vi "Get_Current_Scan_server.vi"(0 "Desired Channels":string[](array[string])) -> (1 "Ch Description Array":T1[](array[typedef]) {"Duty" format="%016b"; "D" format="%#_5g"; "C" format="%#_5g"; "B" format="%#_5g"; "A" format="%#_5g"}, 2 "String values":string[](array[string]), 3 "Numerical Values":dbl[](array[numeric]) format="%.2f")   [LabVIEW 2020]
uses:
  ADAM Client/Sub VIs/ADAM Controls/Ch_description_ADAM.ctl
  ADAM Client/Sub VIs/ADAM Controls/Module_type_ADAM.ctl
  ADAM Client/Sub VIs/ADAM Controls/Function_ADAM.ctl
  ADAM Client/Sub VIs/ADAM Controls/Channel_State.ctl
  ADAM Client/Sub VIs/ADAM Controls/Calib_type_ADAM.ctl
  ADAM Client/Sub VIs/ADAM Controls/Address.ctl
  ADAM_Global.vi
  Sub VI's/Channel_Description_Global.vi
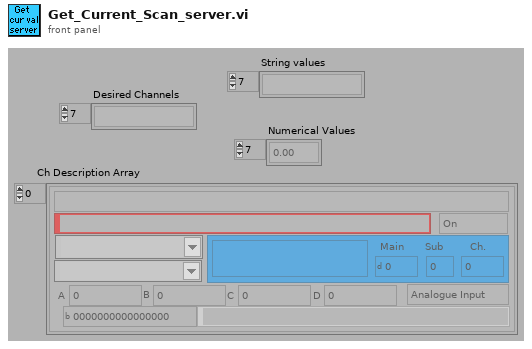
[diagram p1: front panel]
types:
  T1 = typedef "Ch_description_ADAM.ctl" = cluster{"Ch Name":string, "Type":T2, "Function":T3, "Ch State":T4, "Calibration type":T5, "A":dbl, "B":dbl, "C":dbl, "D":dbl, "Comments":string, "Address":T6, "String":string, "Duty":u16}
  T2 = typedef "Module_type_ADAM.ctl" = string
  T3 = typedef "Function_ADAM.ctl" = enum16{"Analogue Input", "Digital Input", "Event counter", "Event rate", "Analogue Output", "Digital Output", "Relay Output"}
  T4 = typedef "Channel_State.ctl" = enum16{"On", "Off", "Always On", "Always Off"}
  T5 = typedef "Calib_type_ADAM.ctl" = string
  T6 = typedef "Address.ctl" = cluster{"Main":i32, "Ch.":i32, "Sub":i32, "Port Name":string}
  T7 = typedef "Update_scan_value.ctl" = cluster{"Channel Name":string, "New Value":dbl}
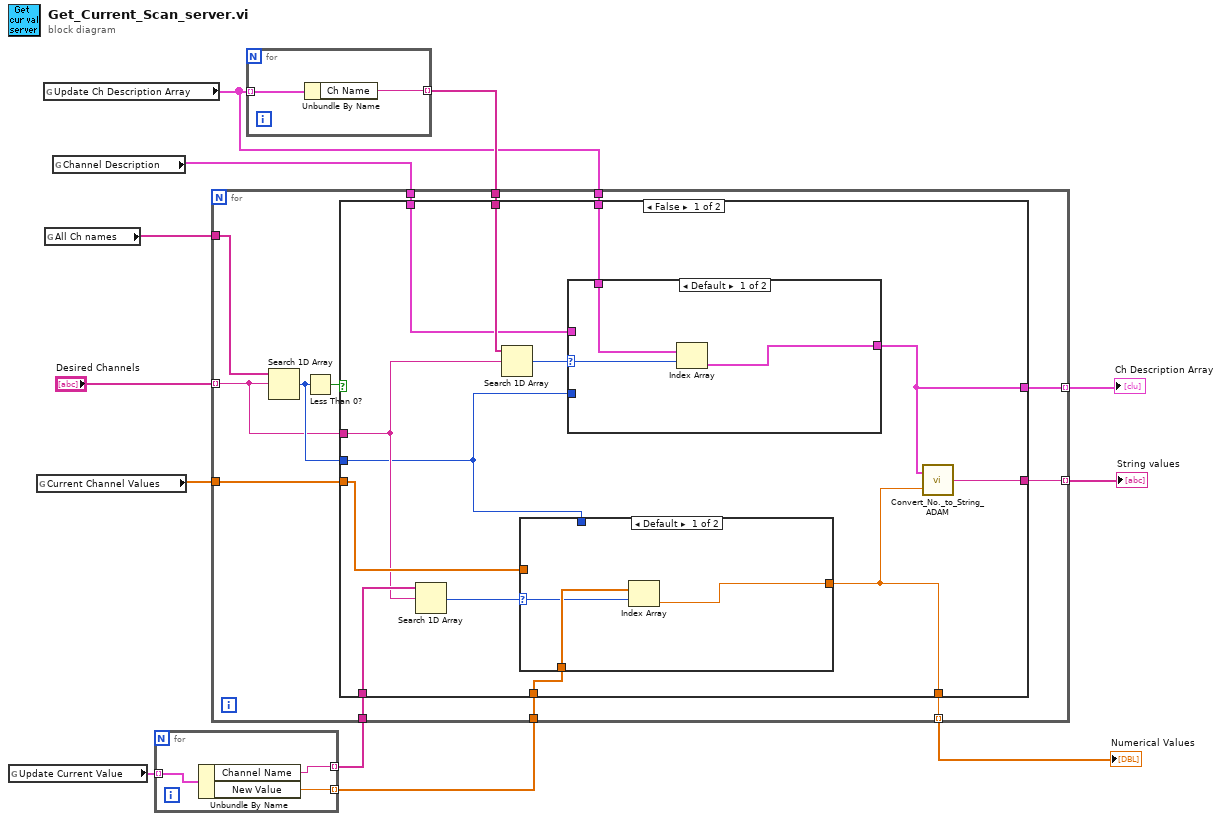
[diagram p0: block diagram]
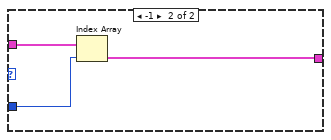
[diagram p2: hidden frame]
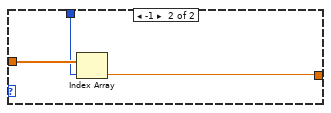
[diagram p3: hidden frame]
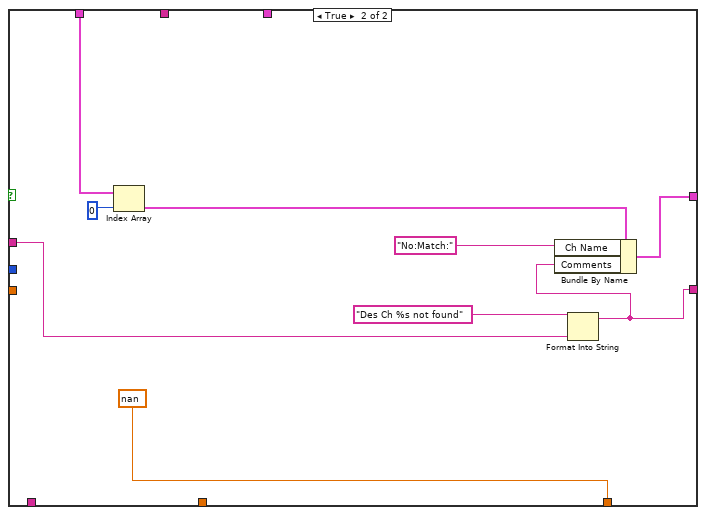
[diagram p4: hidden frame]
diagram:
  n1 = global read "ADAM_Global.vi" "Update Current Value"() -> (w5:T7[])
  n2 = global read "ADAM_Global.vi" "Current Channel Values"() -> (w11:dbl[])
  n3 = global read "ADAM_Global.vi" "Update Ch Description Array"() -> (w1:T1[])
  n4 = global read "ADAM_Global.vi" "All Ch names"() -> (w12:string[])
  n5 = global read "Channel_Description_Global.vi" "Channel Description"() -> (w6:T1[])
  n6 = for {
    tunnel: w5 -> [w15] mode=indexing
    tunnel: [w14] -> w4 mode=indexing
    tunnel: [w13] -> w3 mode=indexing
    n7 = Unbundle By Name(w15) -> ("Channel Name"=w14:string, "New Value"=w13:dbl)
  }
  n8 = for {
    tunnel: w1 -> [w17] mode=indexing
    tunnel: [w16] -> w2 mode=indexing
    n9 = Unbundle By Name(w17) -> ("Ch Name"=w16:string)
  }
  n10 = for {
    tunnel: "Desired Channels" -> [w22] mode=indexing
    tunnel: w12 -> [w30]
    tunnel: [w28] -> w10 mode=indexing
    tunnel: w11 -> [w26]
    tunnel: w6 -> [w25]
    tunnel: [w24] -> w9 mode=indexing
    tunnel: [w23] -> w7 mode=indexing
    tunnel: w4 -> [w21]
    tunnel: w3 -> [w20]
    tunnel: w2 -> [w19]
    tunnel: w1 -> [w18]
    n11 = Search 1D Array(1D array=w30, element=w22) -> (index of element=w27:i32)  [unwired: 1 out]
    n12 = Less Than 0?(x=w27) -> (x < 0?=w29:bool)
    n13 = case shown="False" w29 {
      tunnel: [w43 w56] -> w28
      tunnel: w27 -> [w33 _]
      tunnel: w26 -> [w40 _]
      tunnel: w25 -> [w34 w63]
      tunnel: [w39 nan] -> w24
      tunnel: [w31 w61] -> w23
      tunnel: w22 -> [w35 w58]
      tunnel: w21 -> [w42 _]
      tunnel: w20 -> [w38 _]
      tunnel: w19 -> [w36 _]
      tunnel: w18 -> [w32 _]
      frame False {
        n14 = Search 1D Array(1D array=w42, element=w35) -> (index of element=w41:i32)  [unwired: 1 out]
        n15 = Search 1D Array(1D array=w36, element=w35) -> (index of element=w37:i32)  [unwired: 1 out]
        n16 = case shown="Default" w41 {
          selector: w41 -> [w51 _]
          tunnel: w40 -> [_ w55]
          tunnel: w33 -> [_ w54]
          tunnel: [w50 w53] -> w39
          tunnel: w38 -> [w52 _]
          frame Default {
            n17 = Index Array(array=w52, index=w51) -> (element=w50:dbl)
          }
          frame -1 {
            n18 = Index Array(array=w55, index=w54) -> (element=w53:dbl)
          }
        }
        n19 = case shown="Default" w37 {
          selector: w37 -> [w46 _]
          tunnel: [w45 w49] -> w31
          tunnel: w34 -> [_ w48]
          tunnel: w33 -> [_ w47]
          tunnel: w32 -> [w44 _]
          frame Default {
            n20 = Index Array(array=w44, index=w46) -> (element=w45:T1)
          }
          frame -1 {
            n21 = Index Array(array=w48, index=w47) -> (element=w49:T1)
          }
        }
        n22 = call "Convert_No._to_String_ADAM.vi"("Input number"=w39, "Ch Description"=w31) -> ("Output sting"=w43:string)
      }
      frame True {
        n23 = Index Array(array=w63, index=0 ("Index")) -> (element=w62:T1)
        n24 = Format Into String(format string="Des Ch %s not found", w58) -> (resulting string=w56:string)  [unwired: 2 in, 1 out]
        n25 = Bundle By Name(cluster=w62, "Ch Name"="No:Match:", "Comments"=w56) -> (w61:T1)
      }
    }
  }
  "String values" <- w10
  "Numerical Values" <- w9
  "Ch Description Array" <- w7
